vi "Build NS String.vi"(10 "Previous Namespaces":string, 11 "Namespace name":string) -> (3 "New Namespace string":string)   [LabVIEW 2018, in "Path and String Processing.lvlib"]
uses:
  Path and String Processing.lvlib
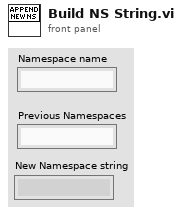
[diagram p1: front panel]
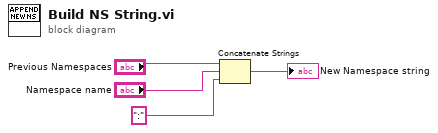
[diagram p0: block diagram]
diagram:
  n1 = Concatenate Strings("Previous Namespaces", "Namespace name", ":") -> (→"New Namespace string":string)
